vi "Write Measurement Configuration.vi"(8 "error in (no error)":errorcluster, 10 "Measurement Configuration":T1={"Function"=enum."2-Wire Resistance", " Manual Resolution"=enum."6.5", "Frequency Source"=enum."AC Voltage", "Auto Range"=enum."ON"}, 11 "Agilent 3458A in":refnum<class "Agilent 3458A.lvclass">) -> (0 "error out":errorcluster, 3 "Agilent 3458A out":refnum<class "Agilent 3458A.lvclass">)   [LabVIEW 2011, in "Agilent 3458A.lvclass"]
uses:
  Agilent 3458A.lvclass
  Measurement Configuration.ctl
  Agilent 3458A.lvclass/Agilent 3458A.ctl
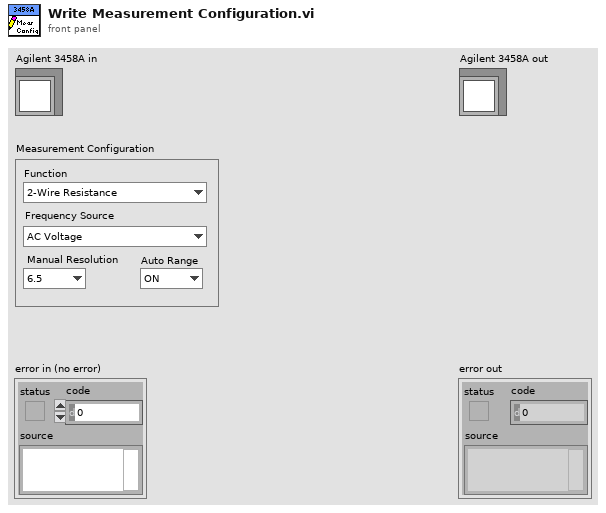
[diagram p1: front panel]
types:
  T1 = typedef "Agilent 3458A.lvclass/Measurement Configuration.ctl" = cluster{"Function":enum16{"DC Voltage", "AC Voltage", "AC + DC Voltage", "DC Current", "AC Current", "AC + DC Current", "2-Wire Resistance", "4-Wire Resistance", "Frequency", "Period", "Direct Sampling DC", "Direct Sampling AC", "Sub-Sampling DC", "Sub-Sampling AC"}, " Manual Resolution":enum16{"4.5", "5.5", "6.5", "7.5", "8.5"}, "Frequency Source":enum16{"AC + DC Current", "AC + DC Voltage", "AC Current", "AC Voltage"}, "Auto Range":enum16{"OFF", "ON", "ONCE"}}
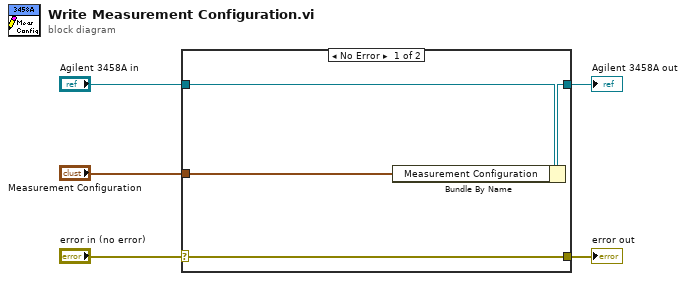
[diagram p0: block diagram]
diagram:
  n1 = case shown="No Error" "error in (no error)" {
    selector: "error in (no error)" -> [w9 w10]
    tunnel: [w9 w10] -> w4
    tunnel: [w7 w11] -> w2
    tunnel: "Agilent 3458A in" -> [w8 w11]
    tunnel: "Measurement Configuration" -> [w6 _]
    frame No Error {
      n2 = Bundle By Name(cluster=w8, "Measurement Configuration"=w6) -> (w7:refnum<class "Agilent 3458A.lvclass">)
    }
    frame Error {
    }
  }
  "error out" <- w4
  "Agilent 3458A out" <- w2
